vi "Read Waveform.vi"(8 "error in (no error)":errorcluster {"code" format="%.0x"}, 11 "VISA Resource Name":refnum<visa-resource-name>) -> (0 "error out":errorcluster {"code" format="%.0x"}, 1 "x increment":dbl caption="x Increment" format="%^.2e", 2 "initial x":dbl caption="Initial x" format="%^.2e", 3 "VISA Resource Name Out":refnum<visa-resource-name>, 4 "waveform array":dbl[](array[numeric]) caption="Waveform Array" format="%.2f", 5 "actual points":u32 caption="Actual Points")   [LabVIEW 2011, in "Agilent 546XX Series.lvlib"]
doc: "This VI initiates an acquisition on the channels that you enable with the ag546xx Configure Channel VI. It then waits for the acquisition to complete, and returns the waveform for the channel you specify. You call the ag546xx Fetch Waveform VI to obtain the waveforms for each of the remaining enabled channels without initiating another acquisition.\n\nNotes:\n\n(1) After this VI executes, each element in the Waveform Array is either a voltage or a value indicating that the oscilloscope could not sample a voltage."
uses:
  Agilent 546XX Series.lvlib
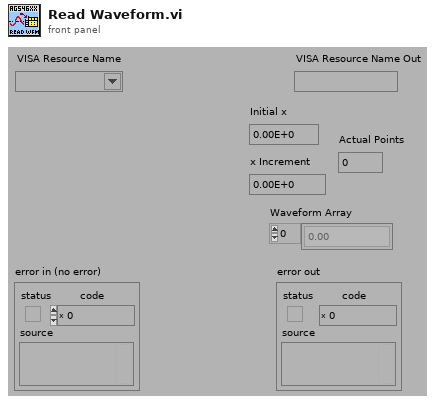
[diagram p1: front panel]
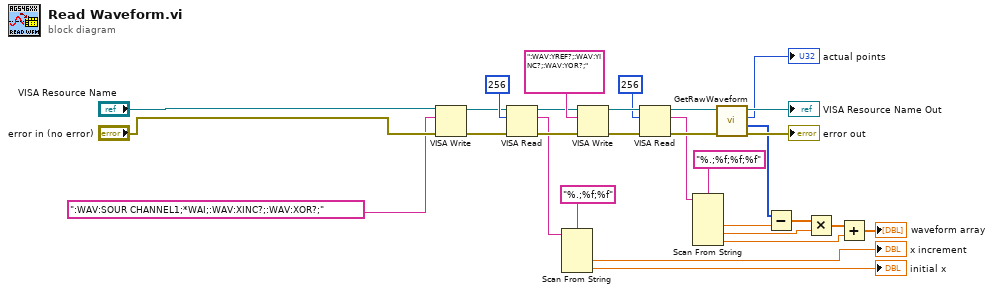
[diagram p0: block diagram]
diagram:
  n1 = VISA Write(VISA resource name="VISA Resource Name", write buffer=":WAV:SOUR CHANNEL1;*WAI;:WAV:XINC?;:WAV:XOR?;", error in (no error)="error in (no error)") -> (VISA resource name out=w11:refnum<visa-resource-name>, error out=w10:errorcluster)  [unwired: 1 out]
  n2 = VISA Read(VISA resource name=w11, byte count=u32 256, error in (no error)=w10) -> (VISA resource name out=w9:refnum<visa-resource-name>, read buffer=w7:string, error out=w8:errorcluster)  [unwired: 1 out]
  n3 = Scan From String(format string="%.;%f;%f", input string=w7) -> (output 1=→"x increment":dbl, output 2=→"initial x":dbl)  [unwired: 4 in, 3 out]
  n4 = VISA Write(VISA resource name=w9, write buffer=":WAV:YREF?;:WAV:YINC?;:WAV:YOR?;", error in (no error)=w8) -> (VISA resource name out=w30:refnum<visa-resource-name>, error out=w29:errorcluster)  [unwired: 1 out]
  n5 = VISA Read(VISA resource name=w30, byte count=u32 256, error in (no error)=w29) -> (VISA resource name out=w28:refnum<visa-resource-name>, read buffer=w22:string, error out=w27:errorcluster)  [unwired: 1 out]
  n6 = Scan From String(format string="%.;%f;%f;%f", input string=w22) -> (output 1=w20:dbl, output 2=w18:dbl, output 3=w16:dbl)  [unwired: 5 in, 3 out]
  n7 = call "GetRawWaveform.vi"("error in"=w27, "VISA Resource Name"=w28) -> ("error out"=→"error out":errorcluster, "Waveform Array"=w14:u32[], "Number of Points"=→"actual points":u32, "VISA Resource Name Out"=→"VISA Resource Name Out":refnum<visa-resource-name>)  [unwired: 5 in, 1 out]
  n8 = Subtract(x=w14, y=w20) -> (x-y=w19:dbl[])
  n9 = Multiply(x=w19, y=w18) -> (x*y=w17:dbl[])
  n10 = Add(x=w17, y=w16) -> (x+y=→"waveform array":dbl[])
